vi "Assign Value.vi"(8 "error in (no error)":errorcluster, 10 "Assigned Value":refnum<class "Abs_Value.lvclass">, 11 "Abs_Time in":refnum<class "Abs_Time 1D.lvclass">) -> (0 "error out":errorcluster, 3 "Abs_Time out":refnum<class "Abs_Time 1D.lvclass">)   [LabVIEW 2021, in "Abs_Time 1D.lvclass"]
uses:
  Abs_Time 1D.lvclass
  Value/Abs_Value.lvclass
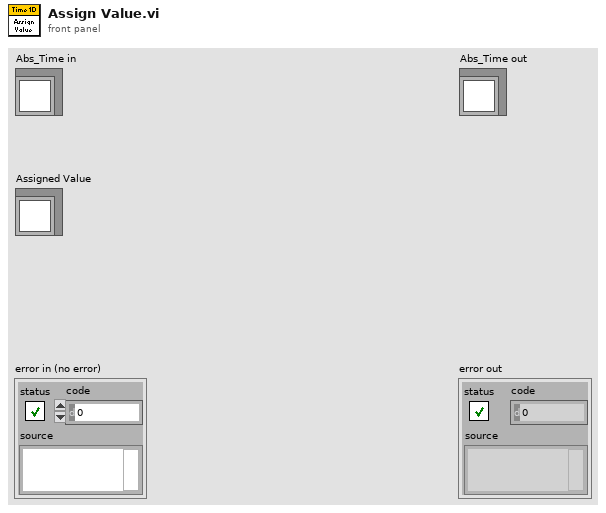
[diagram p1: front panel]
types:
  T1 = typedef "Abs_Time 1D.lvclass/Type.ctl" = timestamp[]
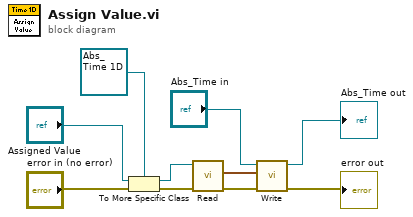
[diagram p0: block diagram]
diagram:
  n1 = To More Specific Class(target class=refnum<class "Abs_Time 1D.lvclass"> refnum ("Abs_Time.lvclass"), reference="Assigned Value", error in="error in (no error)") -> (specific class reference=w6:refnum<class "Abs_Time 1D.lvclass">, error out=w7:errorcluster)
  n2 = call-dynamic "Read.vi"("error in (no error)"=w7, "Double Float.lvclass_340760 in"=w6) -> ("error out"=w5:errorcluster, "Value"=w3:T1)  [unwired: 7 in, 1 out]
  n3 = call-dynamic "Write.vi"("error in (no error)"=w5, "Value"=w3, "Double Float.lvclass_340760 in"="Abs_Time in") -> ("error out"=→"error out":errorcluster, "Double Float.lvclass_340760 out"=→"Abs_Time out":refnum<class "Abs_Time 1D.lvclass">)  [unwired: 7 in]
